vi "Debug Shooter.vi"(1 "% output Shooter":dbl(slide) scale=0.0..1.0, 2 "Target RPM":dbl(slide) scale=0.0..10000.0, 3 "Switch mode":bool, 4 "Enable":bool) -> ()   [LabVIEW 2016]
uses:
  <vilib>/Rock Robotics/WPI/ThirdParty/CanMotor/TalonSRX/WPI_CANTalonSRX_APIFeedbackSelect.ctl
  <vilib>/Rock Robotics/WPI/ThirdParty/CanMotor/TalonSRX/WPI_CANTalonSRX_APIControlMode.ctl
panel:
  in  "Shooter PIDF":T1={"P"=0.2425, "I"=0.0001, "D"=0.0002, "F"=0.0, "I Zone"=0.0, "Ramp Rate"=1.2}
  out "Use Speed":bool
  in  "Swirly %":dbl(slide)=0.8 scale=0.0..1.0
  in  "Feeder %":dbl(slide)=0.9 scale=0.0..1.0
  in  "Reverse Closed-Loop Output":bool
  in  "Reverse Feedback Sensor":bool
  out "Motor output Plot":cluster{"Applied Throttle":dbl}(graph)
  out "Speed Closed Loop Plots":cluster{dbl, "Sensor Velocity":dbl}(graph)
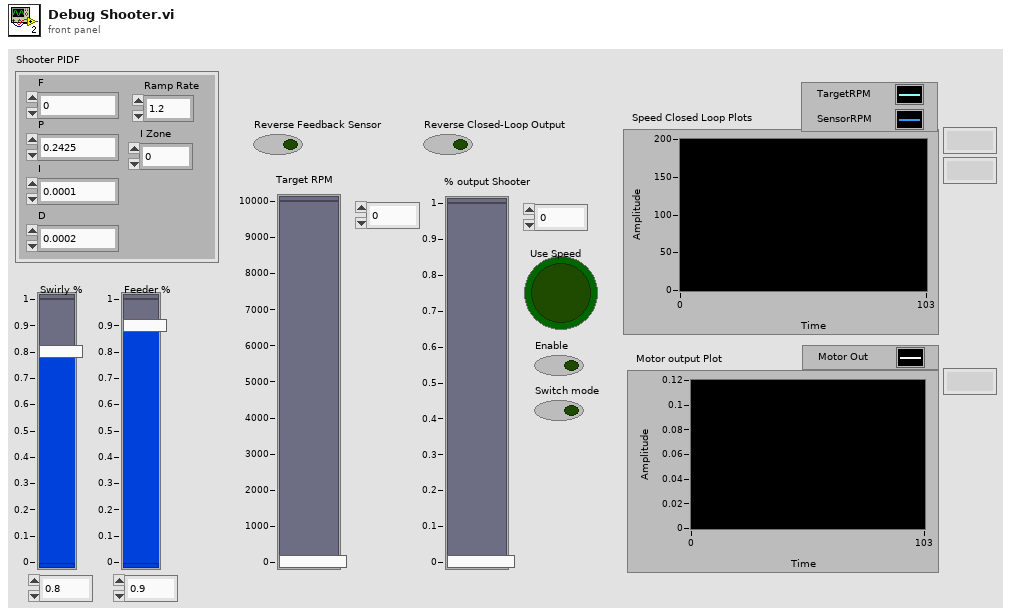
[diagram p1: front panel]
types:
  T1 = cluster{"P":dbl, "I":dbl, "D":dbl, "F":dbl, "I Zone":dbl, "Ramp Rate":dbl}
  T2 = typedef "WPI_CANTalonSRX_APIFeedbackSelect.ctl" = enum16{"Digital Quadrature Encoder", "Analog Potentiometer", "Analog Encoder", "Count on Quad-A (Rising-Edge)", "Count on Quad-A (Falling-Edge)", "CTR Magnetic Enc (Absolute)", "CTR Magnetic Enc (Relative)", "Pulse Width"}
  T3 = typedef "WPI_MotorControlDeviceRef.ctl" = cluster{"DeviceStatus":errorcluster, "Type":T4, "PWM":cluster{"PWM Channel":T5, "DeadBand":T6}, "CAN":cluster{"Device Number":u8, "SetOutput VI Ref":variant, "GetOutput VI Ref":variant, "Enable VI Ref":variant, "Disable VI Ref":variant, "Data":variant}, "Invert":bool}
  T4 = typedef "WPI_MotorControlType.ctl" = enum16{"PWM", "CAN"}
  T5 = typedef "FPGA_DIOPWMChannel.ctl" = enum8{"PWM 0", "PWM 1", "PWM 2", "PWM 3", "PWM 4", "PWM 5", "PWM 6", "PWM 7", "PWM 8", "PWM 9", "PWM MXP 0", "PWM MXP 1", "PWM MXP 2", "PWM MXP 3", "PWM MXP 4", "PWM MXP 5", "PWM MXP 6", "PWM MXP 7", "PWM MXP 8", "PWM MXP 9", "Invalid"}
  T6 = typedef "WPI_PWMDeadband.ctl" = cluster{"Name":string, "maxPositivePwm":i32, "minPositivePwm":i32, "centerPwm":i32, "maxNegativePwm":i32, "minNegativePwm":i32, "angularRange":u16}
  T7 = typedef "WPI_CANTalonSRX_APIControlMode.ctl" = enum8{"Percent VBus", "Speed", "Position", "Slave", "Unchanged / Invalid", "Voltage Compensation", "Current", "Motion Profile", "Motion Magic"}
  T8 = typedef "WPI_CANTalonSRX_GlobalStatus.ctl" = cluster{"Applied Throttle":dbl, "Module Enabled":bool, "CAN Error":errorcluster, "Closed Loop Error":dbl, "Forward Limit Switch Closed":bool, "Reverse Limit Switch Closed":bool, "Sensor Position":dbl, "Sensor Velocity":dbl, "Current":dbl, "Sticky Fault - Over Temp":bool, "Sticky Fault - Under Voltage":bool, "Sticky Fault - Forward Limit":bool, "Sticky Fault - Reverse Limit":bool, "Sticky Fault - Forward Soft Limit":bool, "Sticky Fault - Reverse Soft Limit":bool, "Brake is Enabled":bool, "Encoder Position":dbl, "Encoder Velocity":dbl, "Encoder Index Count":dbl, "Encoder A Pin State":bool, "Encoder B Pin State":bool, "Encoder Index Pin State":bool, "Analog In":dbl, "Analog In Velocity":dbl, "Temperature (C)":dbl, "Battery Voltage":dbl, "Control 5 Is Supported":bool, "Current Profile Slot Select":dbl, "Pos Div 8":bool, "Vel Div 4":bool, "Pulse Width Position":i32, "Pulse Width Velocity":i32, "Pulse Width Rise To Rise (us)":i32, "Pulse Width Rise To Fall (us)":i32, "Mot Prof Active Is Under Run":bool, "Mot Prof Active Has Under Run":bool, "Mot Prof Active Is Last":bool, "Mot Prof Active Velocity Only":bool, "Mot Prof Active Is Valid":bool, "Mot Prof Buffer Is Full":bool, "Mot Prof Active Profile Slot Select":i32, "Mot Prof NextID":i32, "Mot Prof Count":i32, "Mot Prof Active Velocity":dbl, "Mot Prof Active Position":dbl, "Mot Prof Output Enable":i32, "UsageFrame":u32}
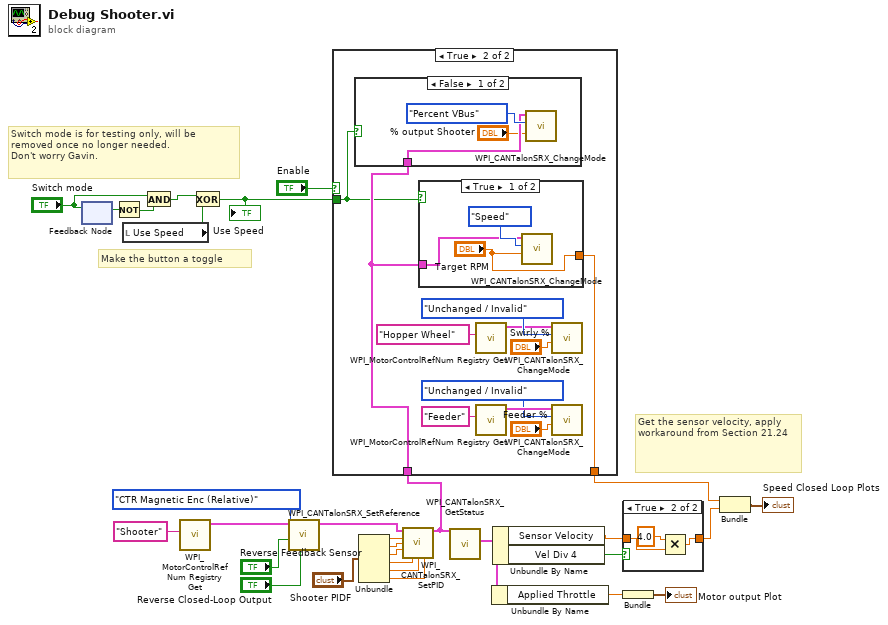
[diagram p0: block diagram]
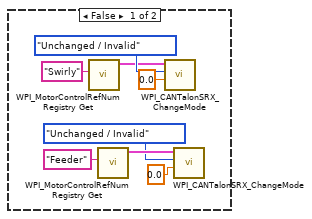
[diagram p2: hidden frame]
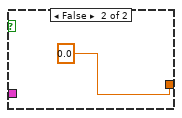
[diagram p4: hidden frame]
diagram:
  # "Switch mode is for testing only, will be \nremoved once no longer needed.\nDon't worry Gavin."
  # "Make the button a toggle"
  # "Get the sensor velocity, apply workaround from Section 21.24"
  n1 = feedback #1() -> (w14:bool)  [unwired: 1 in]
  n2 = feedback-in #1("Switch mode") -> ()
  n3 = Not(x=w14) -> (.not. x?=w13:bool)
  n4 = local read "Use Speed"() -> (w10:bool)
  n5 = And(x="Switch mode", y=w13) -> (x .and. y?=w11:bool)
  n6 = call <vilib>:"WPI_MotorControlRefNum Registry Get.vi"("refnum name"="Shooter") -> ("MotorControlDevRef"=w25:T3)  [unwired: 9 in, 1 out]
  n7 = Exclusive Or(1:w10, 2:w11) -> (0:w12:bool)
  "Use Speed" <- w12
  n8 = call <vilib>:"WPI_CANTalonSRX_SetReference.vi"("Reverse Closed-Loop Output"="Reverse Closed-Loop Output", "Reverse Feedback Sensor"="Reverse Feedback Sensor", "Feedback Reference"=WPI_CANTalonSRX_APIFeedbackSelect."CTR Magnetic Enc (Relative)" ("Feedback Reference Shooter"), "CAN Talon SRX Ref"=w25) -> ("CAN Talon SRX Ref"=w24:T3)  [unwired: 6 in, 1 out]
  n9 = Unbundle("Shooter PIDF") -> ("P"=w8:dbl, "I"=w7:dbl, "D"=w6:dbl, "F"=w5:dbl, "I Zone"=w4:dbl, "Ramp Rate"=w3:dbl)
  n10 = call <vilib>:"WPI_CANTalonSRX_SetPID.vi"("CAN Talon SRX Ref"=w24, "P"=w8, "I"=w7, "D"=w6, "F"=w5, "I Zone"=w4, "Ramp Rate"=w3) -> ("CAN Talon SRX Ref"=w21:T3)  [unwired: 7 in, 1 out]
  n11 = case shown="True" "Enable" {
    tunnel: w21 -> [_ w48]
    tunnel: [_ w47] -> w16
    tunnel: w12 -> [_ w46]
    frame False {
      n12 = call <vilib>:"WPI_MotorControlRefNum Registry Get.vi"("refnum name"="Swirly") -> ("MotorControlDevRef"=w32:T3)  [unwired: 9 in, 1 out]
      n13 = call <vilib>:"WPI_MotorControlRefNum Registry Get.vi"("refnum name"="Feeder") -> ("MotorControlDevRef"=w37:T3)  [unwired: 9 in, 1 out]
      n14 = call <vilib>:"WPI_CANTalonSRX_ChangeMode.vi"("Output"=0.0, "Control Mode"=WPI_CANTalonSRX_APIControlMode."Unchanged / Invalid", "CAN Talon SRX Ref"=w32) -> ()  [unwired: 7 in, 2 out]
      n15 = call <vilib>:"WPI_CANTalonSRX_ChangeMode.vi"("Output"=0.0, "Control Mode"=WPI_CANTalonSRX_APIControlMode."Unchanged / Invalid", "CAN Talon SRX Ref"=w37) -> ()  [unwired: 7 in, 2 out]
    }
    frame True {
      n16 = case shown="False" w46 {
        tunnel: w48 -> [w50 _]
        frame False {
          # "When Button1 is released, PercentVoltage"
          n17 = call <vilib>:"WPI_CANTalonSRX_ChangeMode.vi"("Output"="% output Shooter", "Control Mode"=WPI_CANTalonSRX_APIControlMode."Percent VBus", "CAN Talon SRX Ref"=w50) -> ()  [unwired: 7 in, 2 out]
        }
        frame True {
        }
      }
      n18 = case shown="True" w46 {
        tunnel: w48 -> [w53 _]
        tunnel: ["Target RPM" 0.0 ("x")] -> w47
        frame True {
          n19 = call <vilib>:"WPI_CANTalonSRX_ChangeMode.vi"("Output"="Target RPM", "Control Mode"=WPI_CANTalonSRX_APIControlMode."Speed", "CAN Talon SRX Ref"=w53) -> ()  [unwired: 7 in, 2 out]
        }
        frame False {
        }
      }
      n20 = call <vilib>:"WPI_MotorControlRefNum Registry Get.vi"("refnum name"="Hopper Wheel") -> ("MotorControlDevRef"=w38:T3)  [unwired: 9 in, 1 out]
      n21 = call <vilib>:"WPI_MotorControlRefNum Registry Get.vi"("refnum name"="Feeder") -> ("MotorControlDevRef"=w45:T3)  [unwired: 9 in, 1 out]
      n22 = call <vilib>:"WPI_CANTalonSRX_ChangeMode.vi"("Output"="Swirly %", "Control Mode"=WPI_CANTalonSRX_APIControlMode."Unchanged / Invalid", "CAN Talon SRX Ref"=w38) -> ()  [unwired: 7 in, 2 out]
      n23 = call <vilib>:"WPI_CANTalonSRX_ChangeMode.vi"("Output"="Feeder %", "Control Mode"=WPI_CANTalonSRX_APIControlMode."Unchanged / Invalid", "CAN Talon SRX Ref"=w45) -> ()  [unwired: 7 in, 2 out]
    }
  }
  n24 = call <vilib>:"WPI_CANTalonSRX_GetStatus.vi"("CAN Talon SRX Ref"=w21) -> ("Talon SRX Status"=w22:T8)  [unwired: 8 in, 2 out]
  n25 = Unbundle By Name(w22) -> ("Applied Throttle"=w19:dbl)
  n26 = Unbundle By Name(w22) -> ("Sensor Velocity"=w27:dbl, "Vel Div 4"=w26:bool)
  n27 = case shown="True" w26 {
    tunnel: [w56 w58] -> w15
    tunnel: w27 -> [w56 w57]
    frame False {
    }
    frame True {
      n28 = Multiply(x=4.0, y=w57) -> (x*y=w58:dbl)
    }
  }
  n29 = Bundle("Applied Throttle"=w19) -> (→"Motor output Plot":cluster{"Applied Throttle":dbl})  [unwired: 1 in]
  n30 = Bundle("x"=w16, "Sensor Velocity"=w15) -> (→"Speed Closed Loop Plots":cluster{"x":dbl, "Sensor Velocity":dbl})  [unwired: 1 in]
